vi "compare channel list to typedefs.vi"(8 "error in":errorcluster, 11 "fixed channel configuration":refnum<class "fixed channel configuration.lvclass">) -> (0 "error out":errorcluster, 3 "configured channels out":refnum<class "TBM channel.lvclass">[](array[class]))   [LabVIEW 2013, in "fixed channel configuration.lvclass"]
uses:
  fixed channel configuration.lvclass
  <vilib>/NI/Tag Bus Module Framework/channel/TBM channel.lvclass
  fixed channel configuration.lvclass/fixed channel configuration.ctl
  <vilib>/NI/Tag Bus/tag/tag descriptor.lvclass/tag descriptor.ctl
  <vilib>/NI/Tag Bus/tag/tag descriptor.lvclass
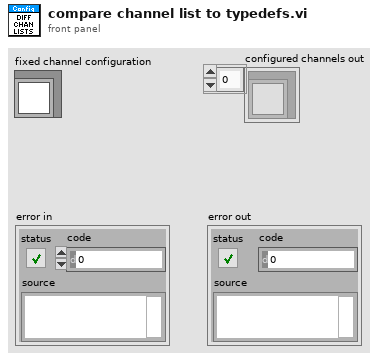
[diagram p1: front panel]
types:
  T1 = typedef "tag bus.lvlib/tag descriptor.lvclass/Data Type.ctl" = enum16{"Double", "Single", "I64", "I32", "I16", "I8", "U64", "U32", "U16", "U8", "Boolean", "String", "Array of Double", "Array of Single", "Array of I64", "Array of I32", "Array of I16", "Array of I8", "Array of U64", "Array of U32", "Array of U16", "Array of U8", "Array of Boolean", "Array of String"}
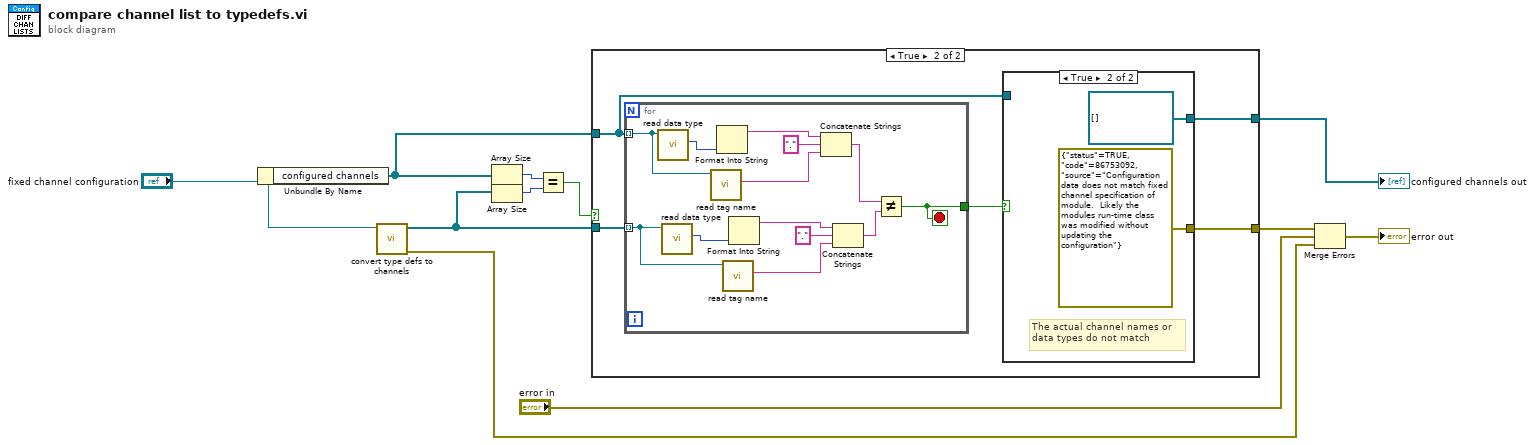
[diagram p0: block diagram]
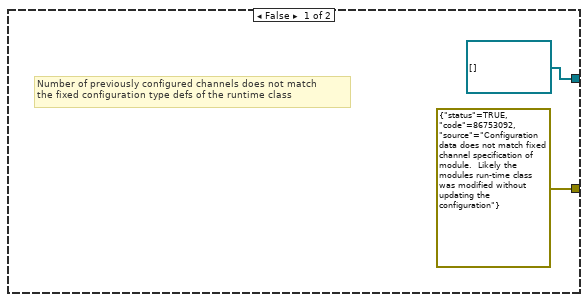
[diagram p2: hidden frame]
diagram:
  n1 = Unbundle By Name("fixed channel configuration") -> ("configured channels"=w1:refnum<class "TBM channel.lvclass">[])
  n2 = call "convert type defs to channels.vi"("fixed channel configuration"="fixed channel configuration") -> ("error out"=w3:errorcluster, "Array out"=w4:refnum<class "TBM channel.lvclass">[])  [unwired: 9 in]
  n3 = Array Size(array=w1) -> (size(s)=w8:i32)
  n4 = Array Size(array=w4) -> (size(s)=w9:i32)
  n5 = Equal?(x=w8, y=w9) -> (x = y?=w7:bool)
  n6 = case shown="True" w7 {
    tunnel: w1 -> [_ w16]
    tunnel: [errorcluster {"status"=TRUE, "code"=86753092, "source"="Configuration data does not match fixed channel specification of module.  Likely the modules run-time class was modified without updating the configuration"} ("error constant") w17] -> w10
    tunnel: [refnum<class "TBM channel.lvclass">[] [] ("configured channels") w15] -> w11
    tunnel: w4 -> [_ w14]
    frame False {
      # "Number of previously configured channels does not match\nthe fixed configuration type defs of the runtime class"
    }
    frame True {
      n7 = for {
        tunnel: w16 -> [w31] mode=indexing
        tunnel: [w30] -> w18
        tunnel: w14 -> [w23] mode=indexing
        stop <- w30 stop-if-true
        n8 = call <vilib>:"read data type.vi"("system tag in"=w31) -> ("data type"=w34:T1)  [unwired: 8 in, 2 out]
        n9 = call <vilib>:"read data type.vi"("system tag in"=w23) -> ("data type"=w24:T1)  [unwired: 8 in, 2 out]
        n10 = call <vilib>:"read tag name.vi"("system tag in"=w31) -> ("name"=w33:string)  [unwired: 8 in, 2 out]
        n11 = Format Into String(w34) -> (resulting string=w32:string)  [unwired: 3 in, 1 out]
        n12 = call <vilib>:"read tag name.vi"("system tag in"=w23) -> ("name"=w25:string)  [unwired: 8 in, 2 out]
        n13 = Format Into String(w24) -> (resulting string=w26:string)  [unwired: 3 in, 1 out]
        n14 = Concatenate Strings(w32, "." ("resulting string"), w33) -> (w28:string)
        n15 = Concatenate Strings(w26, "." ("resulting string"), w25) -> (w22:string)
        n16 = Not Equal?(x=w28, y=w22) -> (x != y?=w30:bool)
      }
      n17 = case shown="True" w18 {
        tunnel: [_ errorcluster {"status"=TRUE, "code"=86753092, "source"="Configuration data does not match fixed channel specification of module.  Likely the modules run-time class was modified without updating the configuration"} ("error constant")] -> w17
        tunnel: w16 -> [w19 _]
        tunnel: [w19 refnum<class "TBM channel.lvclass">[] [] ("configured channels")] -> w15
        frame False {
        }
        frame True {
          # "The actual channel names or\ndata types do not match"
        }
      }
    }
  }
  "configured channels out" <- w11
  n18 = Merge Errors(w10, "error in", w3) -> (→"error out":errorcluster)
